vi "De_noise.vi"(6 "u(t)":dbl) -> (2 "u(t)2":dbl)   [LabVIEW 2018]
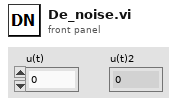
[diagram p1: front panel]
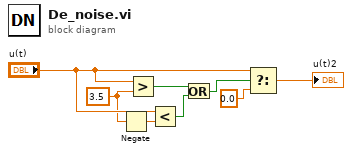
[diagram p0: block diagram]
diagram:
  w4 = 3.5
  n1 = Negate(x=w4) -> (-x=w5:dbl)
  n2 = Greater?(x="u(t)", y=w4) -> (0:w7:bool)
  n3 = Less?(x="u(t)", y=w5) -> (x < y?=w8:bool)
  n4 = Or(x=w7, y=w8) -> (x .or. y?=w3:bool)
  n5 = Select(t="u(t)", s=w3, f=0.0) -> (s? t:f=→"u(t)2":dbl)
